vi "Test_telecommande.vi"() -> ()   [LabVIEW 2011]
uses:
  <vilib>/DAQmx/write.llb/DAQmx Write (Digital Bool 1Line 1Point).vi
  <vilib>/DAQmx/miscellaneous.llb/DAQmx Fill In Error Info.vi
panel:
  in  "Ouest":bool
  in  "Sud":bool
  in  "Nord":bool
  in  "Est":bool
  in  "stop":bool
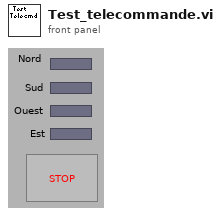
[diagram p1: front panel]
types:
  T1 = cluster{"North Task":refnum<k21>, "West Task":refnum<k21>, "South Task":refnum<k21>, "East Task":refnum<k21>}
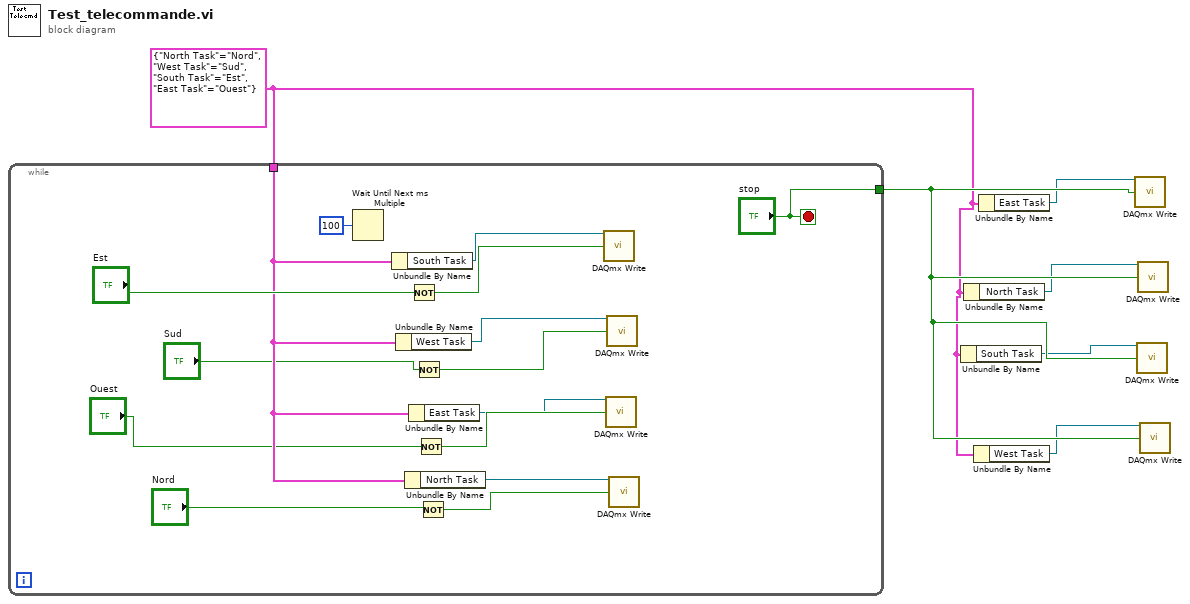
[diagram p0: block diagram]
diagram:
  w1 = T1 {"North Task"="Nord", "West Task"="Sud", "South Task"="Est", "East Task"="Ouest"} ("TaskCluster")
  n1 = while {
    tunnel: w1 -> [w17]
    tunnel: ["stop"] -> w6
    stop <- "stop" stop-if-true
    n2 = Wait Until Next ms Multiple(millisecond multiple=u32 100 ("n millisecondes")) -> ()  [unwired: 1 out]
    n3 = Unbundle By Name(w17) -> ("South Task"=w21:refnum<k21>)
    n4 = Unbundle By Name(w17) -> ("West Task"=w16:refnum<k21>)
    n5 = Unbundle By Name(w17) -> ("North Task"=w8:refnum<k21>)
    n6 = Not(x="Est") -> (.not. x?=w19:bool)
    n7 = Unbundle By Name(w17) -> ("East Task"=w11:refnum<k21>)
    n8 = Not(x="Sud") -> (.not. x?=w15:bool)
    n9 = Not(x="Ouest") -> (.not. x?=w12:bool)
    n10 = Not(x="Nord") -> (.not. x?=w9:bool)
    n11 = call-poly <vilib>:"DAQmx Write.vi"("task/channels in"=w21, "data"=w19) -> ()  [unwired: 11 in, 3 out]
    n12 = call-poly <vilib>:"DAQmx Write.vi"("task/channels in"=w11, "data"=w12) -> ()  [unwired: 11 in, 3 out]
    n13 = call-poly <vilib>:"DAQmx Write.vi"("task/channels in"=w16, "data"=w15) -> ()  [unwired: 11 in, 3 out]
    n14 = call-poly <vilib>:"DAQmx Write.vi"("task/channels in"=w8, "data"=w9) -> ()  [unwired: 11 in, 3 out]
  }
  n15 = Unbundle By Name(w1) -> ("South Task"=w4:refnum<k21>)
  n16 = Unbundle By Name(w1) -> ("North Task"=w3:refnum<k21>)
  n17 = Unbundle By Name(w1) -> ("West Task"=w5:refnum<k21>)
  n18 = Unbundle By Name(w1) -> ("East Task"=w2:refnum<k21>)
  n19 = call-poly <vilib>:"DAQmx Write.vi"("task/channels in"=w2, "data"=w6) -> ()  [unwired: 11 in, 3 out]
  n20 = call-poly <vilib>:"DAQmx Write.vi"("task/channels in"=w4, "data"=w6) -> ()  [unwired: 11 in, 3 out]
  n21 = call-poly <vilib>:"DAQmx Write.vi"("task/channels in"=w3, "data"=w6) -> ()  [unwired: 11 in, 3 out]
  n22 = call-poly <vilib>:"DAQmx Write.vi"("task/channels in"=w5, "data"=w6) -> ()  [unwired: 11 in, 3 out]
